vi "Read Analog Input.vi"(7 "Unit Address (1)":i16=1, 8 "error in (no error)":errorcluster {"code" format="%.0x"}, 10 "Analog Input (1)":i16=1, 11 "VISA resource name":refnum<visa-resource-name>) -> (0 "error out":errorcluster {"code" format="%.0x"}, 2 "Value":dbl format="%.2f", 3 "VISA resource name out":refnum<visa-resource-name>)   [LabVIEW 2010]
doc: "This VI is used to read Analog Input value."
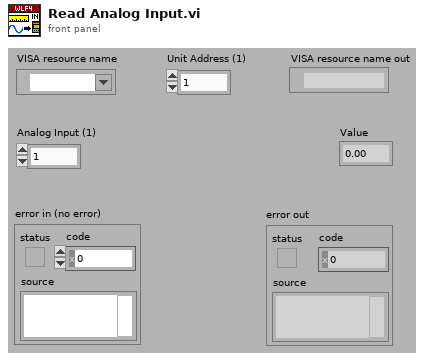
[diagram p1: front panel]
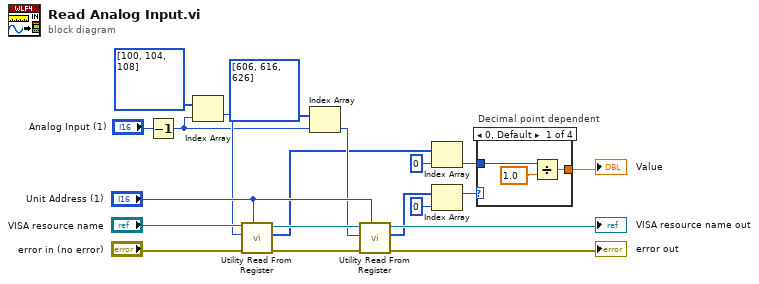
[diagram p0: block diagram]
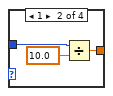
[diagram p2: hidden frame]
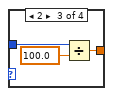
[diagram p3: hidden frame]
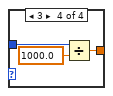
[diagram p4: hidden frame]
diagram:
  # "Decimal point dependent"
  n1 = Decrement(x="Analog Input (1)") -> (x-1=w6:i16)
  n2 = Index Array(array=i32[] [100, 104, 108], index=w6) -> (element=w8:i32)
  n3 = call "Utility Read From Register.vi"("Unit Address (1)"="Unit Address (1)", "error in (no error)"="error in (no error)", "Register Address (0)"=w8, "VISA resource name"="VISA resource name") -> ("error out"=w10:errorcluster, "Data"=w3:i16[], "VISA resource name out"=w9:refnum<visa-resource-name>)  [unwired: 5 in]
  n4 = Index Array(array=i32[] [606, 616, 626], index=w6) -> (element=w5:i32)
  n5 = call "Utility Read From Register.vi"("Unit Address (1)"="Unit Address (1)", "error in (no error)"=w10, "Register Address (0)"=w5, "VISA resource name"=w9) -> ("error out"=→"error out":errorcluster, "Data"=w17:i16[], "VISA resource name out"=→"VISA resource name out":refnum<visa-resource-name>)  [unwired: 5 in]
  n6 = Index Array(array=w3, index=0) -> (element=w2:i16)
  n7 = Index Array(array=w17, index=0) -> (element=w16:i16)
  n8 = case shown="0, Default" w16 {
    tunnel: [w22 w25 w28 w31] -> w1
    tunnel: w2 -> [w21 w24 w27 w30]
    frame 0, Default {
      n9 = Divide(x=w21, y=1.0) -> (x/y=w22:dbl)
    }
    frame 1 {
      n10 = Divide(x=w24, y=10.0) -> (x/y=w25:dbl)
    }
    frame 2 {
      n11 = Divide(x=w27, y=100.0) -> (x/y=w28:dbl)
    }
    frame 3 {
      n12 = Divide(x=w30, y=1000.0) -> (x/y=w31:dbl)
    }
  }
  "Value" <- w1
